vi "myRIO v1.0 Reset FPGA.vi"(8 "error in (no error)":errorcluster, 11 "Generic FPGA Reference in":T1) -> (0 "error out":errorcluster, 3 "Generic FPGA Reference out":T1)   [LabVIEW 2021]
uses:
  <vilib>/myRIO/Common/Instrument Driver Framework/Utilities/typedefs/Generic FPGA Reference.ctl
  <vilib>/FPGAPlugInAG/Dynamic/niLvFpga_Reset_Dynamic.vi
  <vilib>/FPGAPlugInAG/Dynamic/niLvFpga_Run_Dynamic.vi
  <vilib>/rvi/interface/nirviMethod/nirviMethod.xnode
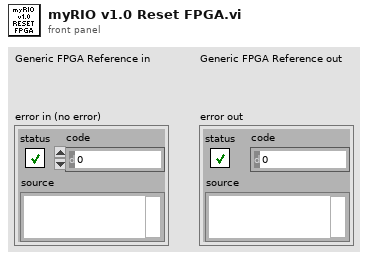
[diagram p1: front panel]
types:
  T1 = typedef "Generic FPGA Reference.ctl" = refnum<k20>
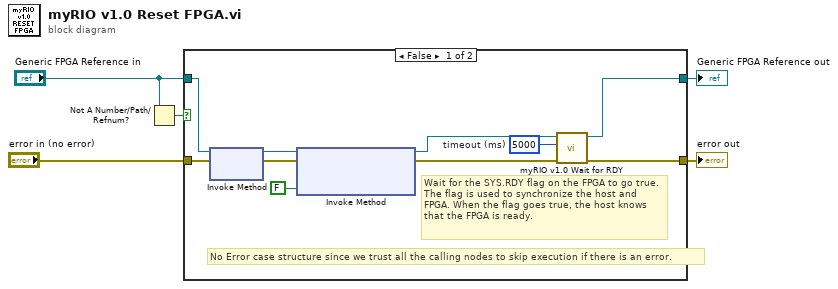
[diagram p0: block diagram]
diagram:
  n1 = Not A Number/Path/Refnum?(number/path/refnum="Generic FPGA Reference in") -> (NaN/Path/Refnum?=w3:bool)
  n2 = case shown="False" w3 {
    tunnel: "Generic FPGA Reference in" -> [w12 w17]
    tunnel: [w14 w17] -> w5
    tunnel: [w13 w16] -> w4
    tunnel: "error in (no error)" -> [w11 w16]
    frame False {
      w15 = 5000  # timeout (ms)
      # "Wait for the SYS.RDY flag on the FPGA to go true. The flag is used to synchronize the host and FPGA. When the flag goes true, the host knows that the FPGA is ready."
      # "No Error case structure since we trust all the calling nodes to skip execution if there is an error."
      n3 = xnode "Invoke Method"("FPGA VI Reference In"=w12, "error in"=w11) -> ("FPGA VI Reference Out"=w10:T1, "error out"=w9:errorcluster)
      n4 = xnode "Invoke Method"("FPGA VI Reference In"=w10, "error in"=w9, "Wait Until Done (F)"=FALSE) -> ("FPGA VI Reference Out"=w7:T1, "error out"=w6:errorcluster)
      n5 = call <vilib>:"myRIO v1.0 Wait for RDY.vi"("error in (no error)"=w6, "timeout (ms)"=w15, "Generic FPGA Reference in"=w7) -> ("error out"=w13:errorcluster, "Generic FPGA Reference out"=w14:T1)  [unwired: 7 in]
    }
    frame True {
    }
  }
  "Generic FPGA Reference out" <- w5
  "error out" <- w4
